vi "Wrap Image metadata.vi"(11 "image metadata":T1[](array[typedef])) -> (1 "element":T3, 2 "Numeric":i32, 3 "total bytes":u32)   [LabVIEW 2025, in "Automotive Vision.lvclass"]
doc: "Converts data to make the calling vi cleaner."
uses:
  Automotive Vision.lvclass
  Automotive Vision.lvclass/Automotive Vision.ctl
  <instrlib>/FlexRIO/CSI-2/v2/Common/Types/LLP Data Type.ctl
  <instrlib>/FlexRIO/CSI-2/v2/Common/NI CSI-2 API Common v2.lvlib
  deps/NI148X/Getting Started/FPGA/Common/Types/Image Metadata.ctl
  deps/NI148X/Getting Started/FPGA/Common/GettingStarted_Common_148X_FPGA.lvlib
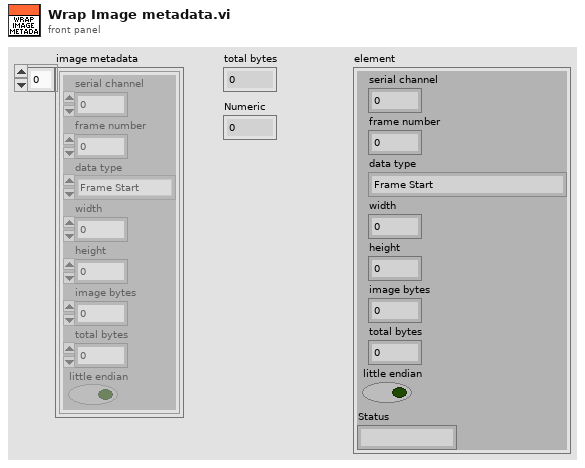
[diagram p1: front panel]
types:
  T1 = typedef "GettingStarted_Common_148X_FPGA.lvlib/Image Metadata.ctl" = cluster{"serial channel":fxp<+,3,3>, "frame number":u16, "data type":T2, "width":u16, "height":u16, "image bytes":u32, "total bytes":u32, "little endian":bool}
  T2 = typedef "NI CSI-2 API Common v2.lvlib/LLP Data Type.ctl" = enum8{"Frame Start", "Frame End", "Line Start", "Line End", "End of Transmission", "Reserved 0", "Reserved 1", "Reserved 2", "Generic Short Packet 1", "Generic Short Packet 2", "Generic Short Packet 3", "Generic Short Packet 4", "Generic Short Packet 5", "Generic Short Packet 6", "Generic Short Packet 7", "Generic Short Packet 8", "Null", "Blanking Data", "Embedded 8-bit non Image Data", "Generic Long Packet 1", "Generic Long Packet 2", "Generic Long Packet 3", "Generic Long Packet 4", "Reserved 3", "YUV420 8-bit", "YUV420 10-bit", "Legacy YUV420 8-bit", "Reserved 4", "YUV420 8-bit Chroma Shifted", "YUV420 10-bit Chroma Shifted", "YUV422 8-bit", "YUV422 10-bit", "RGB444", "RGB555", "RGB565", "RGB666", "RGB888", "Reserved 5", "Reserved 6", "RAW 24", "RAW 6", "RAW 7", "RAW 8", "RAW 10", "RAW 12", "RAW 14", "RAW 16", "RAW 20", "User Defined 8-bit Data 1", "User Defined 8-bit Data 2", "User Defined 8-bit Data 3", "User Defined 8-bit Data 4", "User Defined 8-bit Data 5", "User Defined 8-bit Data 6", "User Defined 8-bit Data 7", "User Defined 8-bit Data 8", "USL Command", "Reserved 7", "Reserved 8", "Reserved 9", "Reserved 10", "Reserved 11", "Reserved 12", "LRTE EPD Spacer"}
  T3 = cluster{"serial channel":fxp<+,3,3>, "frame number":u16, "data type":T2, "width":u16, "height":u16, "image bytes":u32, "total bytes":u32, "little endian":bool, "Status":string}
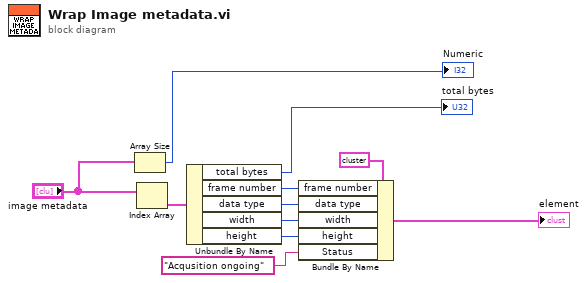
[diagram p0: block diagram]
diagram:
  n1 = Array Size(array="image metadata") -> (size(s)=→"Numeric":i32)
  n2 = Index Array(array="image metadata") -> (element=w4:T1)  [unwired: 1 in]
  n3 = Unbundle By Name(w4) -> ("total bytes"=→"total bytes":u32, "frame number"=w5:u16, "data type"=w6:T2, "width"=w7:u16, "height"=w8:u16)
  n4 = Bundle By Name(cluster=T3 {"serial channel"=0.0, "frame number"=0, "data type"=enum."Frame Start", "width"=0, "height"=0, "image bytes"=0, "total bytes"=0, "little endian"=FALSE, "Status"="Ready for Acquisition"} ("element"), "frame number"=w5, "data type"=w6, "width"=w7, "height"=w8, "Status"="Acqusition ongoing") -> (→"element":T3)
